vi "stepUpDown.vi"(8 "Direction":bool, 9 "Step":i32, 10 "Array":i16[][](array[numeric]), 11 "VISA resource name":refnum<visa-resource-name>) -> (1 "StepNum":i32, 2 "DirectionOut":bool, 3 "StepTime":dbl)   [LabVIEW 2020]
uses:
  <vilib>/NI Modbus.llb/MB Serial Master Query Write Multiple Registers (poly).vi
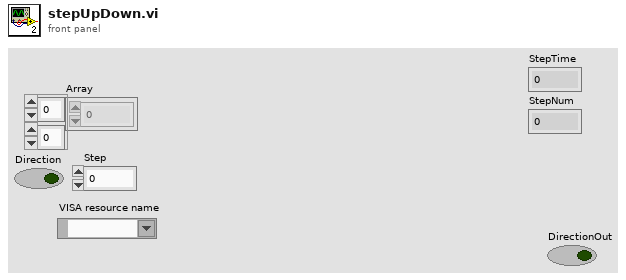
[diagram p1: front panel]
types:
  T1 = cluster{"Mode":enum16{"RTU", "ASCII"}, "Slave Address":u8}
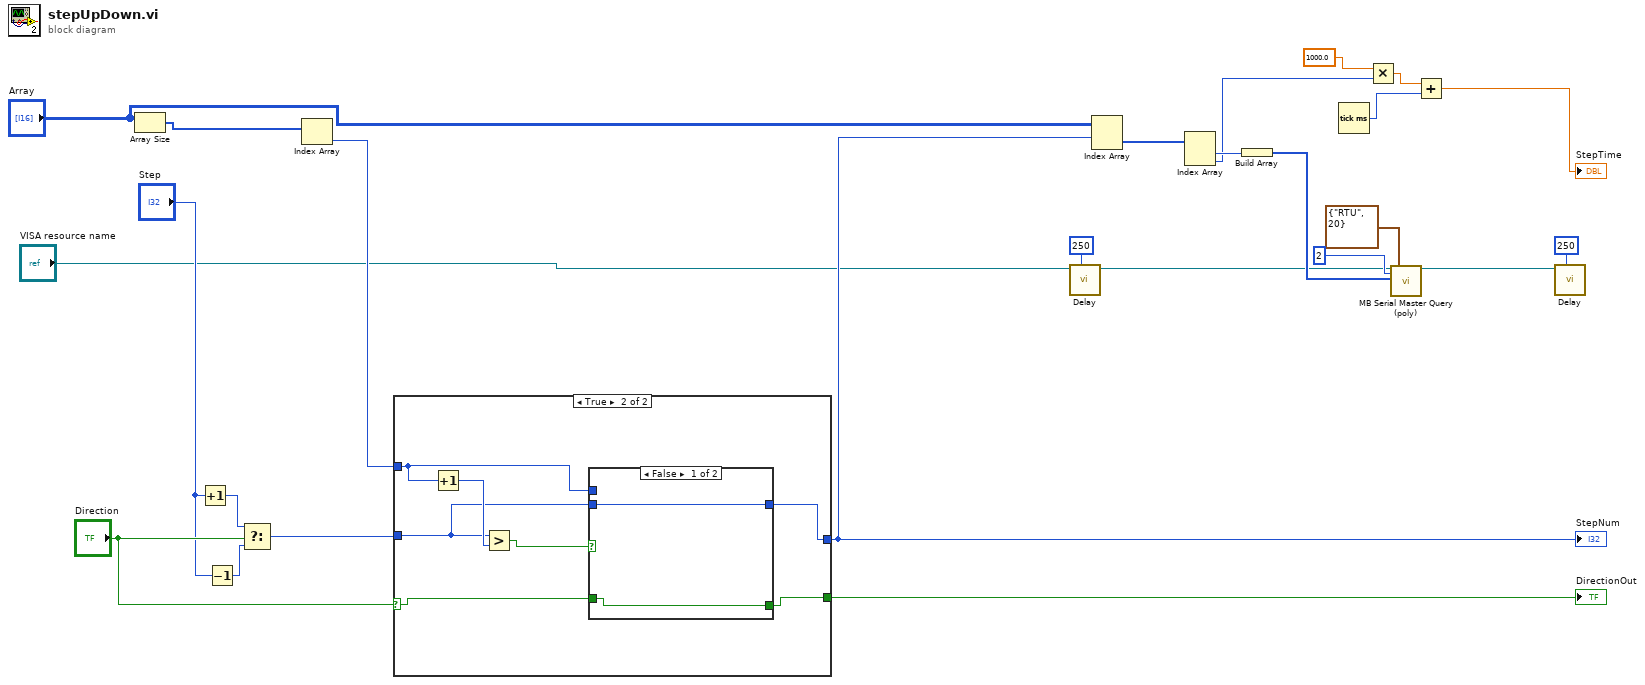
[diagram p0: block diagram]
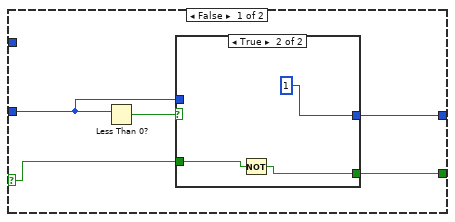
[diagram p2: hidden frame]
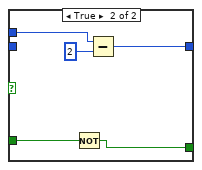
[diagram p4: hidden frame]
diagram:
  n1 = Array Size(array="Array") -> (size(s)=w16:i32[])
  n2 = Increment(x="Step") -> (x+1=w21:i32)
  n3 = Decrement(x="Step") -> (x-1=w20:i32)
  n4 = Select(t=w21, s="Direction", f=w20) -> (s? t:f=w18:i32)
  n5 = Index Array(array=w16) -> (element=w15:i32)  [unwired: 1 in]
  n6 = case shown="True" "Direction" {
    selector: "Direction" -> [w28 w40]
    tunnel: w18 -> [w26 w36]
    tunnel: w15 -> [_ w37]
    tunnel: [w29 w38] -> w14
    tunnel: [w27 w39] -> w11
    frame False {
      n7 = Less Than 0?(x=w26) -> (x < 0?=w30:bool)
      n8 = case shown="True" w30 {
        tunnel: [w31 i16 1 ("t")] -> w29
        tunnel: w28 -> [w32 w34]
        tunnel: [w32 w33] -> w27
        tunnel: w26 -> [w31 _]
        frame False {
        }
        frame True {
          n9 = Not(x=w34) -> (.not. x?=w33:bool)
        }
      }
    }
    frame True {
      n10 = Increment(x=w37) -> (x+1=w42:i32)
      n11 = Greater?(x=w36, y=w42) -> (0:w41:bool)
      n12 = case shown="False" w41 {
        tunnel: [w43 w49] -> w39
        tunnel: w40 -> [w43 w48]
        tunnel: [w44 w46] -> w38
        tunnel: w37 -> [_ w45]
        tunnel: w36 -> [w44 _]
        frame False {
        }
        frame True {
          n13 = Not(x=w48) -> (.not. x?=w49:bool)
          n14 = Subtract(x=w45, y=2) -> (x-y=w46:i32)
        }
      }
    }
  }
  "DirectionOut" <- w11
  "StepNum" <- w14
  n15 = call "Delay.vi"("milliseconds to wait"=u32 250, "VISA Refnum  In"="VISA resource name") -> ("VISA Refnum out"=w3:refnum<visa-resource-name>)  [unwired: 8 in, 1 out]
  n16 = Index Array(array="Array", index (row)=w14) -> (element=w22:i16[])  [unwired: 1 in]
  n17 = Index Array(array=w22) -> (element #1=w13:i16, element #2=w10:i16)  [unwired: 2 in]
  n18 = Build Array(w13) -> (w12:i16[])
  n19 = Tick Count (ms)() -> (millisecond timer value=w7:u32)
  n20 = Multiply(x=1000.0 ("y"), y=w10) -> (x*y=w8:dbl)
  n21 = call-poly <vilib>:"MB Serial Master Query (poly).vi"("VISA resource name"=w3, "Starting Address"=u16 2, "Registers"=w12, "Serial Parameters"=T1 {"Mode"=enum."RTU", "Slave Address"=20}) -> ("VISA resource name out"=w1:refnum<visa-resource-name>)  [unwired: 2 in, 13 out]
  n22 = Add(x=w8, y=w7) -> (x+y=→"StepTime":dbl)
  n23 = call "Delay.vi"("milliseconds to wait"=u32 250, "VISA Refnum  In"=w1) -> ()  [unwired: 8 in, 2 out]
